vi "hyperloop.vi"() -> ()   [LabVIEW 2014]
uses:
  <vilib>/regexp/Match Regular Expression.xnode
panel:
  in  "Tab Control":enum32{"Main Instruments", "Page 2"}(tab)
  out "Velocity (MPH)":dbl(knob) scale=0.0..500.0
  in  "Manual Control":bool
  in  "Emergency Shutoff":bool
  out "Internal Pressure (PSI)":dbl(knob) scale=0.0..200.0 scale format="%#.3g"
  out "Z-pos (feet)":dbl
  out "Y-pos (feet)":dbl
  out "X-pos (feet)":dbl
  out "Tank Pressure (PSI)":dbl(knob) scale=0.0..200.0 scale format="%#.3g"
  out "Yaw (degrees)":dbl
  out "Pitch (degrees)":dbl
  out "Roll (degrees)":dbl
  out "Acceleration (G)":dbl(knob) scale=-2.0..2.0
  out "Temperature (C)":dbl(slide) scale=0.0..200.0 scale format="%#.3g"
  out "Power Consumption (kW)":dbl(slide) scale=0.0..200.0 scale format="%#.3g"
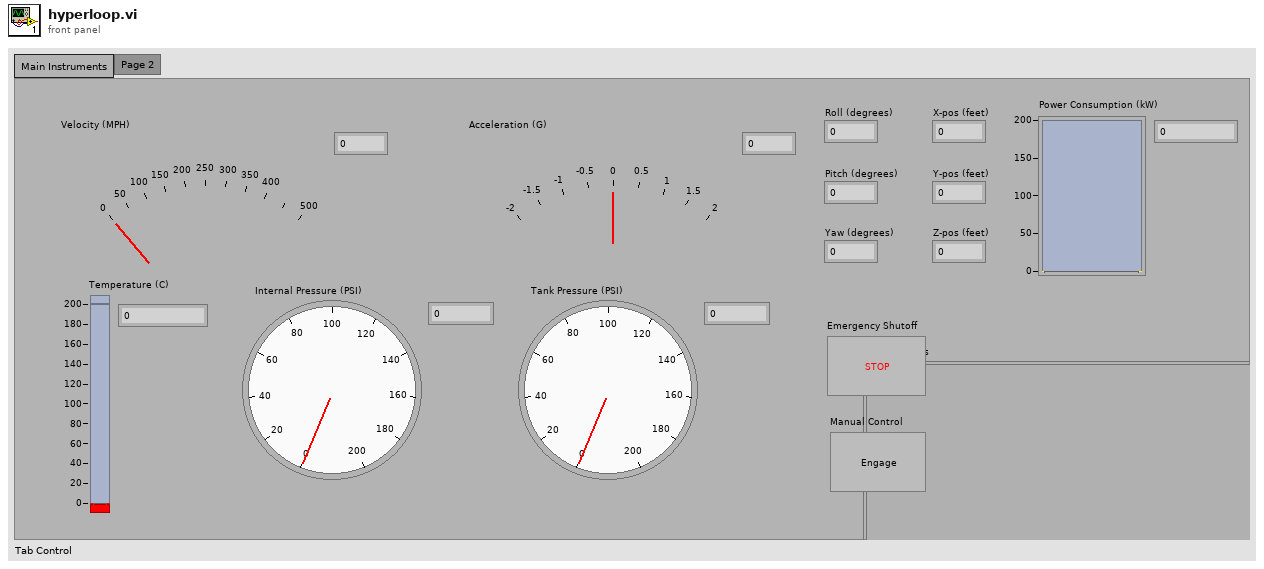
[diagram p1: front panel]
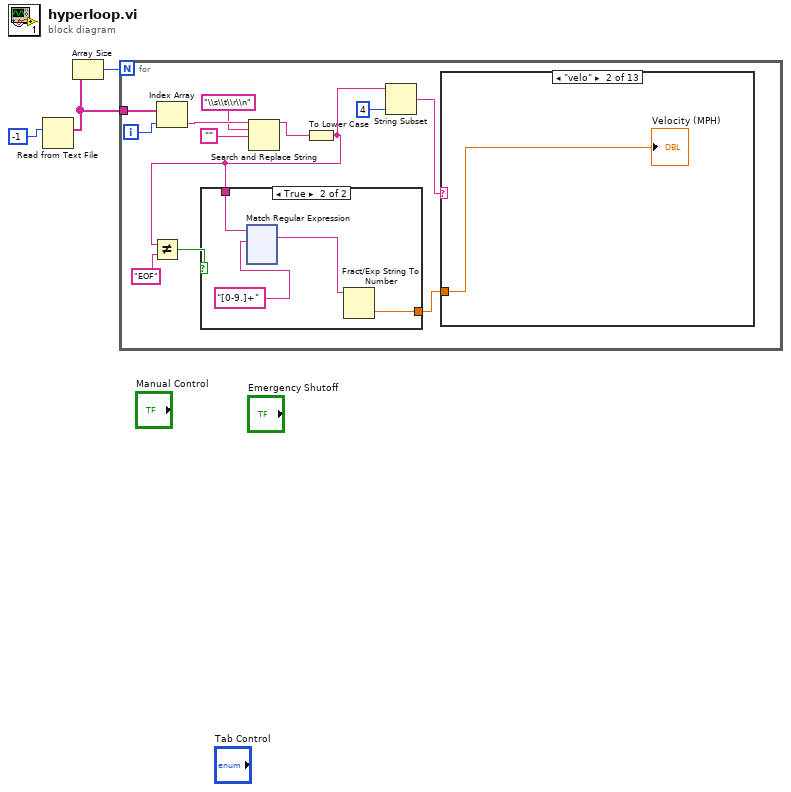
[diagram p0: block diagram]
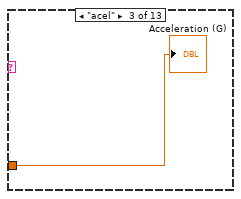
[diagram p4: hidden frame]
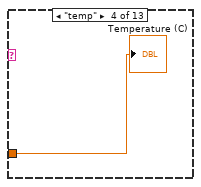
[diagram p5: hidden frame]
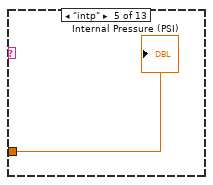
[diagram p6: hidden frame]
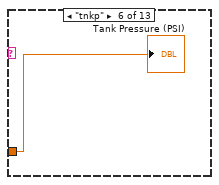
[diagram p7: hidden frame]
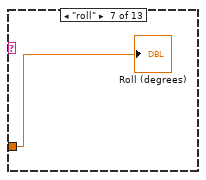
[diagram p8: hidden frame]
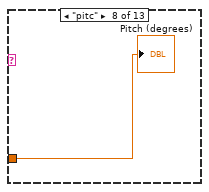
[diagram p9: hidden frame]
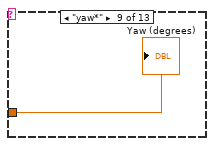
[diagram p10: hidden frame]
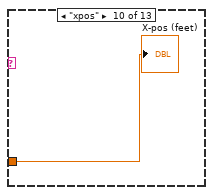
[diagram p11: hidden frame]
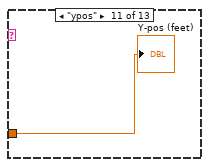
[diagram p12: hidden frame]
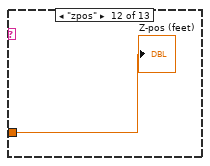
[diagram p13: hidden frame]
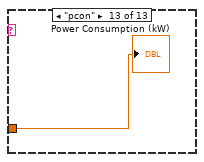
[diagram p14: hidden frame]
diagram:
  n1 = Read from Text File(count=-1) -> (text=w1:string[])  [unwired: 3 in, 3 out]
  n2 = Array Size(array=w1) -> (size(s)=w2:i32)
  n3 = for {
    N: w2 -> [_]
    tunnel: w1 -> [w15]
    i -> [w14]
    n4 = Index Array(array=w15, index=w14) -> (element=w13:string)
    n5 = Search and Replace String(input string=w13, search string="\\s\\t\\r\\n", replace string="") -> (result string=w10:string)  [unwired: 5 in, 3 out]
    n6 = To Lower Case(string=w10) -> (all lower case string=w6:string)
    n7 = Not Equal?(x=w6, y="EOF") -> (x != y?=w5:bool)
    n8 = case shown="True" w5 {
      tunnel: w6 -> [_ w19]
      tunnel: [_ w17] -> w4
      frame False {
      }
      frame True {
        n9 = xnode "Match Regular Expression"("input string"=w19, "regular expression"="[0-9.]+") -> ("whole match"=w16:string)  [unwired: 4 in, 4 out]
        n10 = Fract/Exp String To Number(string=w16) -> (number=w17:dbl)  [unwired: 3 in, 1 out]
      }
    }
    n11 = String Subset(string=w6, length (rest)=4) -> (substring=w8:string)  [unwired: 1 in]
    n12 = case shown="\"velo\"" w8 {
      tunnel: w4 -> [_ w134 w135 w136 w137 w138 w139 w140 w141 w142 w143 w144 w145]
      frame "eof*", Default {
      }
      frame "velo" {
        "Velocity (MPH)" <- w134
      }
      frame "acel" {
        "Acceleration (G)" <- w135
      }
      frame "temp" {
        "Temperature (C)" <- w136
      }
      frame "intp" {
        "Internal Pressure (PSI)" <- w137
      }
      frame "tnkp" {
        "Tank Pressure (PSI)" <- w138
      }
      frame "roll" {
        "Roll (degrees)" <- w139
      }
      frame "pitc" {
        "Pitch (degrees)" <- w140
      }
      frame "yaw*" {
        "Yaw (degrees)" <- w141
      }
      frame "xpos" {
        "X-pos (feet)" <- w142
      }
      frame "ypos" {
        "Y-pos (feet)" <- w143
      }
      frame "zpos" {
        "Z-pos (feet)" <- w144
      }
      frame "pcon" {
        "Power Consumption (kW)" <- w145
      }
    }
  }
